vi "BuildWorker Controller Tester.vi"() -> ()   [LabVIEW 2017]
uses:
  Classes/BuildWorker Basics/BuildWorker Basics.lvclass
panel:
  in  "Show":bool=TRUE
  in  "Port":i32=4545
  in  "remove":bool
  in  "launch":bool
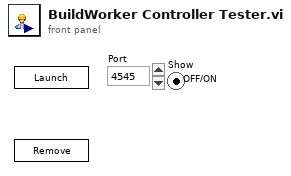
[diagram p1: front panel]
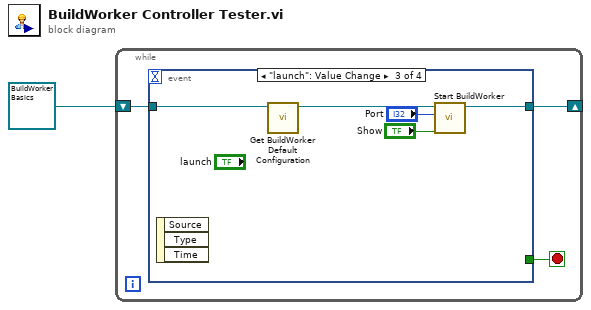
[diagram p0: block diagram]
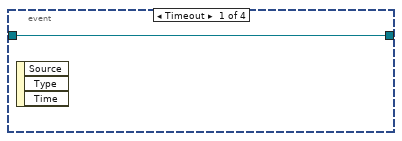
[diagram p2: hidden frame]
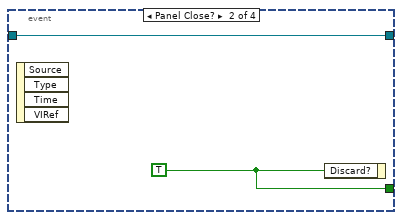
[diagram p3: hidden frame]
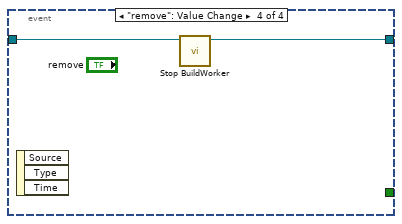
[diagram p4: hidden frame]
diagram:
  n1 = while {
    shift-right: [w2] -> _
    shift-left: refnum<class "BuildWorker Basics.lvclass"> refnum ("BuildWorker Controller.lvlib:BuildWorker Basics.lvclass") -> [w3]
    stop <- w4 stop-if-true
    n2 = event shown="[2] \"launch\": Value Change" {
      selector: _ -> [_ _ _ _]
      dyn-events: _ -> [_ _ _ _]
      timeout: _ -> [_ _ _ _]
      tunnel: [_ w7 _ _] -> w4
      tunnel: w3 -> [w5 w6 w9 w14]
      tunnel: [w5 w6 w10 w13] -> w2
      event Timeout {
        n3 = event-data() -> ()  [unwired: 1 in, 3 out]
      }
      event Panel Close? {
        w7 = TRUE ("Discard?")
        n4 = event-data() -> ()  [unwired: 1 in, 4 out]
        n5 = event-data("Discard?"=w7) -> ()  [unwired: 1 in, 1 out]
      }
      event "launch": Value Change {
        n6 = event-data() -> ()  [unwired: 1 in, 3 out]
        n7 = call-dynamic "Get BuildWorker Default Configuration.vi"("BuildWorker Basics in"=w9) -> ("BuildWorker Basics out"=w8:refnum<class "BuildWorker Basics.lvclass">)  [unwired: 8 in, 2 out]
        n8 = call-dynamic "Start BuildWorker.vi"("Show"="Show", "Port"="Port", "BuildWorker Basics in"=w8) -> ("BuildWorker Basics out"=w10:refnum<class "BuildWorker Basics.lvclass">)  [unwired: 7 in, 1 out]
      }
      event "remove": Value Change {
        n9 = event-data() -> ()  [unwired: 1 in, 3 out]
        n10 = call-dynamic "Stop BuildWorker.vi"("BuildWorker Basics in"=w14) -> ("BuildWorker Basics out"=w13:refnum<class "BuildWorker Basics.lvclass">)  [unwired: 9 in, 1 out]
      }
    }
  }
